vi "(SubVI) Get Dynamic Pixel Value Range Min and Max.vi"(4 "error in (no error)":errorcluster, 7 "Refnum in":T1) -> (0 "error out":errorcluster, 1 "PixelDynamicRangeMax":dbl, 2 "PixelDynamicRangeMin":dbl, 3 "Refnum out":T1)   [LabVIEW 2014]
uses:
  <vilib>/userdefined/High Color/IMAQdx.ctl
  <resource>/objmgr/imaqdx.rc
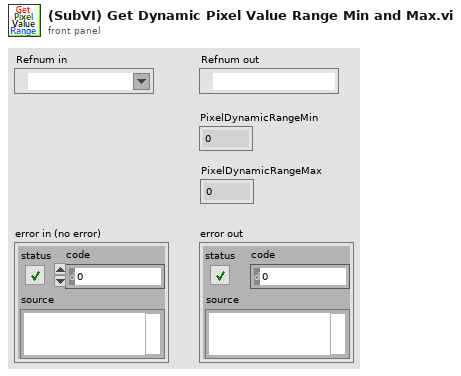
[diagram p1: front panel]
types:
  T1 = typedef "IMAQdx.ctl" = refnum<k21>
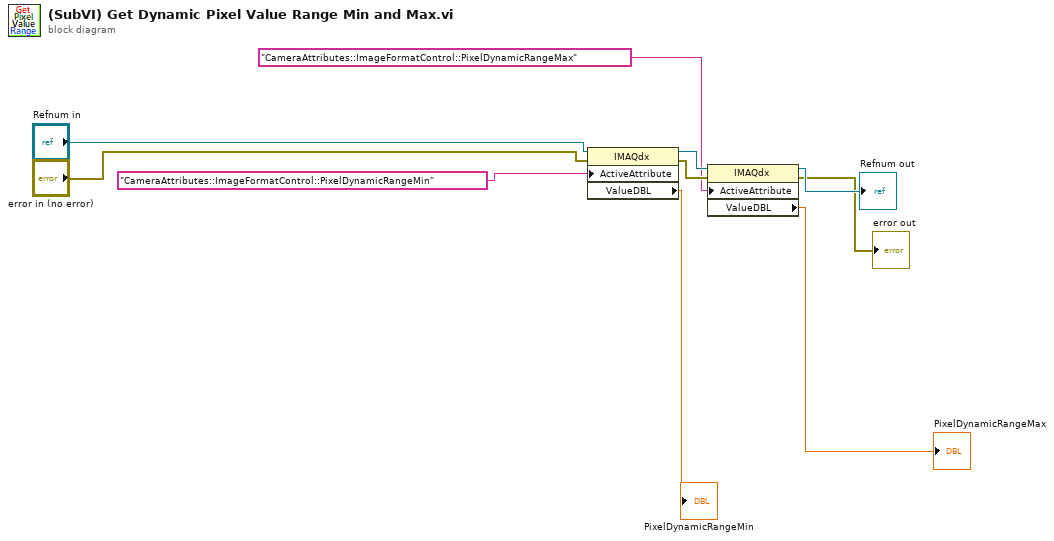
[diagram p0: block diagram]
diagram:
  n1 = property class="IMAQdx"(reference="Refnum in", error in="error in (no error)", "ActiveAttribute"="CameraAttributes::ImageFormatControl::PixelDynamicRangeMin") -> (reference out=w4:T1, error out=w5:errorcluster, "ValueDBL"=→"PixelDynamicRangeMin":dbl)
  n2 = property class="IMAQdx"(reference=w4, error in=w5, "ActiveAttribute"="CameraAttributes::ImageFormatControl::PixelDynamicRangeMax") -> (reference out=→"Refnum out":T1, error out=→"error out":errorcluster, "ValueDBL"=→"PixelDynamicRangeMax":dbl)
